vi "LCR_MEMs Only Beam Control Data.vi"(0 "Channel (0-5)":u32, 1 "Vref (-1: Unchanged)":dbl=-1.0 format="%.3f V", 2 "VISA IN":refnum<visa-resource-name>, 5 "Voltage":dbl format="%.3f V", 11 "Error In":errorcluster, 12 "FPGA":T1) -> (3 "VISA Out":refnum<visa-resource-name>, 4 "Data Out":string, 13 "Cap DBL":dbl, 14 "CAP (fF)":i32, 15 "Error Out":errorcluster)   [LabVIEW 2017]
uses:
  WS_VCAP Driver 1_49/Source/WSVCAP Shell/Type Defs/WSVCAP SHL FPGA Enum.ctl
  WS_VCAP Driver 1_49/Source/WSVCAP Shell/WSVCAP Shell Host Low Level/Host SRL/Host SRL.lvlib
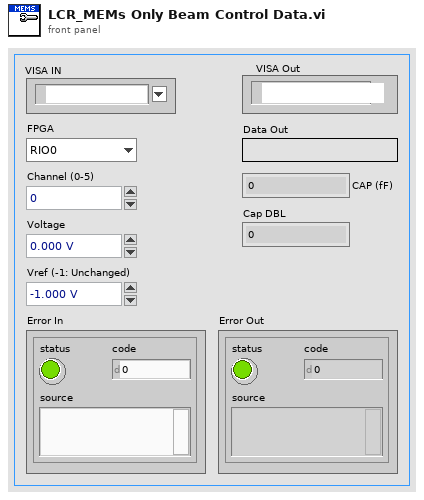
[diagram p1: front panel]
types:
  T1 = typedef "WSVCAP SHL FPGA Enum.ctl" = enum16{"RIO0", "RIO1"}
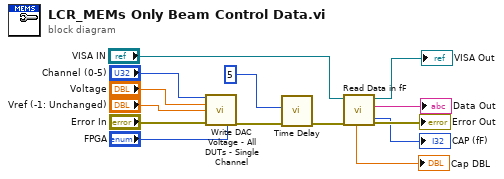
[diagram p0: block diagram]
diagram:
  n1 = call "Write DAC Voltage - All DUTs - Single Channel.vi"("Channel (0-5)"="Channel (0-5)", "Voltage"="Voltage", "Vref (-1: Unchanged)"="Vref (-1: Unchanged)", "error in"="Error In", "FPGA"="FPGA") -> ("error out"=w4:errorcluster)  [unwired: 9 in, 1 out]
  n2 = call "Time Delay.vi"("Error In"=w4, "Delay(ms)"=u32 5) -> ("Error Out"=w5:errorcluster)  [unwired: 9 in]
  n3 = call "Read Data in fF.vi"("Error In"=w5, "VISA IN"="VISA IN") -> ("Error Out"=→"Error Out":errorcluster, "Capacitance(fF)"=→"Data Out":string, "VISA Out"=→"VISA Out":refnum<visa-resource-name>, "CAP (fF)"=→"CAP (fF)":i32, "Cap DBL"=→"Cap DBL":dbl)  [unwired: 4 in, 1 out]
